vi "shutDownCamera.vi"(8 "error in (no error)":errorcluster, 10 "Log in":refnum<class "Log.lvclass">, 11 "ICCameraController in":refnum<class "ICCameraController.lvclass">) -> (0 "error out":errorcluster, 2 "Log out":refnum<class "Log.lvclass">, 3 "ICCameraController out":refnum<class "ICCameraController.lvclass">)   [LabVIEW 2009, in "Hardware.lvlib" / "Channels.lvlib" / "ICCameraController.lvclass"]
uses:
  ICCameraController.lvclass
  Tools/Log.lvclass
  ICCameraController.lvclass/ICCameraController.ctl
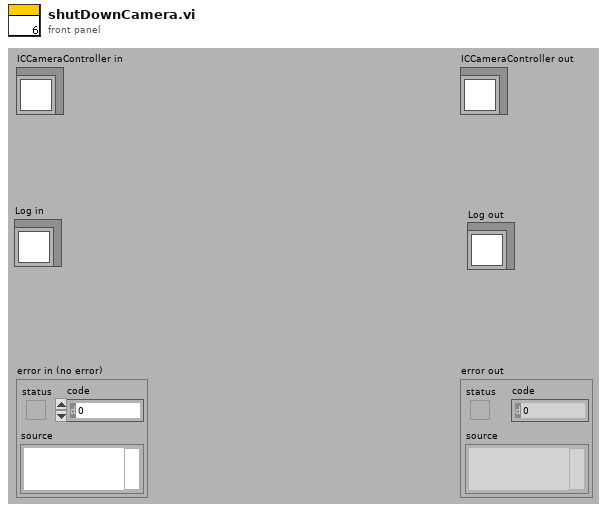
[diagram p1: front panel]
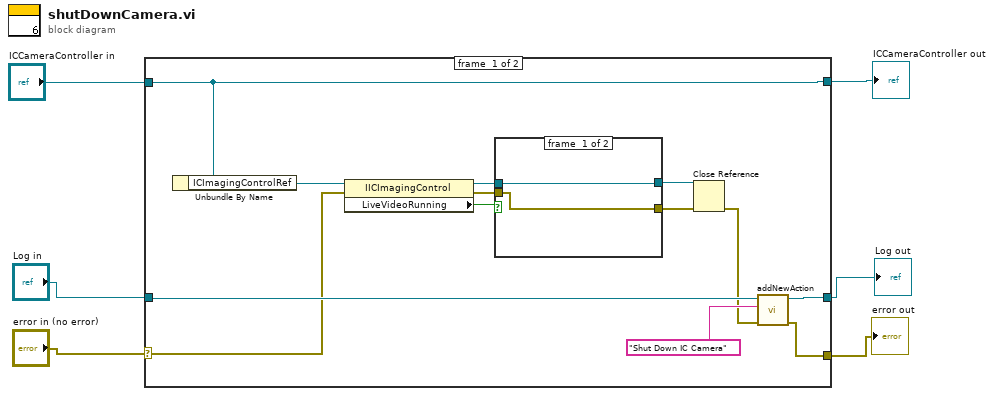
[diagram p0: block diagram]
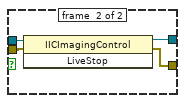
[diagram p2: hidden frame]
diagram:
  n1 = case shown="No Error" "error in (no error)" {
    selector: "error in (no error)" -> [w8 w27]
    tunnel: "Log in" -> [w18 w26]
    tunnel: [w17 w26] -> w4
    tunnel: [w16 w27] -> w3
    tunnel: [w15 w28] -> w2
    tunnel: "ICCameraController in" -> [w15 w28]
    frame #0 {
      n2 = Unbundle By Name(w15) -> ("ICImagingControlRef"=w10:refnum<k7>)
      n3 = property class="IICImagingControl"(reference=w10, error in=w8) -> (reference out=w11:refnum<k7>, error out=w9:errorcluster, "LiveVideoRunning"=w7:bool)
      n4 = case shown="True" w7 {
        tunnel: [w21 w25] -> w14
        tunnel: [w20 w24] -> w13
        tunnel: w11 -> [w21 w23]
        tunnel: w9 -> [w20 w22]
        frame #0 {
        }
        frame #1 {
          n5 = invoke class="IICImagingControl" method="LiveStop"(reference=w23, error in=w22) -> (reference out=w25:refnum<k7>, error out=w24:errorcluster)  [unwired: 1 in, 1 out]
        }
      }
      n6 = Close Reference(reference=w14, error in (no error)=w13) -> (error out=w12:errorcluster)
      n7 = call-dynamic "addNewAction.vi"("error in (no error)"=w12, "newAction"="Shut Down IC Camera", "Log in"=w18) -> ("error out"=w16:errorcluster, "Log out"=w17:refnum<class "Log.lvclass">)  [unwired: 7 in]
    }
    frame #1 {
    }
  }
  "error out" <- w3
  "ICCameraController out" <- w2
  "Log out" <- w4
